vi "Write and Read Multiple Registers Response.vi"(8 "error in (no error)":errorcluster, 10 "Modbus data unit in":refnum<class "Modbus Data Unit (PDU).lvclass">) -> (0 "error out":errorcluster, 1 "registers":u16[](array[numeric]), 2 "byte count":u8)   [LabVIEW 2017, in "SubVIs.lvlib" / "Master Function Definition.lvlib"]
doc: "Decodes the response generated by the write and read multiple holding registers function."
uses:
  <vilib>/Modbus/subvis/Data and Functions/Master Function Definition/Master Function Definition.lvlib
  <vilib>/Modbus/subvis/Modbus Data Unit (PDU)/Modbus Data Unit (PDU).lvclass
  <vilib>/Modbus/subvis/SubVIs.lvlib
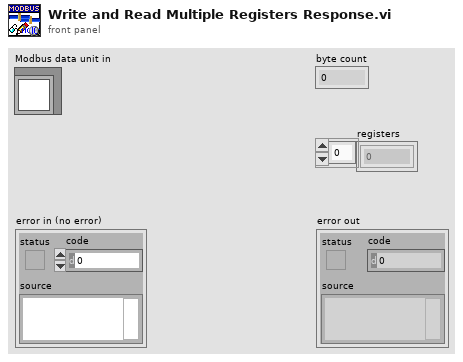
[diagram p1: front panel]
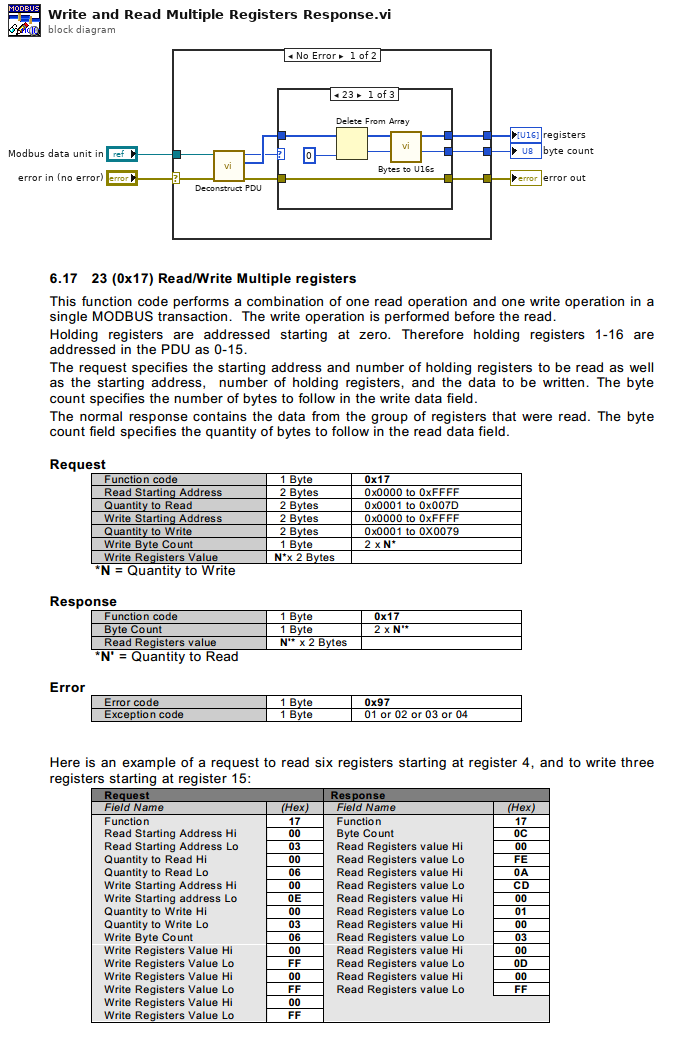
[diagram p0: block diagram]
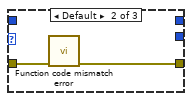
[diagram p2: hidden frame]
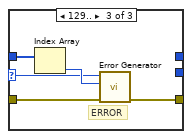
[diagram p3: hidden frame]
diagram:
  n1 = case shown="No Error" "error in (no error)" {
    selector: "error in (no error)" -> [w12 w27]
    tunnel: [w13 w27] -> w4
    tunnel: "Modbus data unit in" -> [w10 _]
    tunnel: [w7 _] -> w2
    tunnel: [w6 _] -> w1
    frame No Error {
      n2 = call <vilib>:"Deconstruct PDU.vi"("error in (no error)"=w12, "Modbus data unit in"=w10) -> ("error out"=w9:errorcluster, "data"=w11:u8[], "function"=w8:u8)  [unwired: 7 in]
      n3 = case shown="23" w8 {
        selector: w8 -> [_ _ w22]
        tunnel: w9 -> [w19 w21 w23]
        tunnel: w11 -> [w16 _ w26]
        tunnel: [w19 w20 w25] -> w13
        tunnel: [w15 _ _] -> w7
        tunnel: [w14 _ _] -> w6
        frame 23 {
          n4 = Delete From Array(array=w16, index=0) -> (deleted portion=w15:u8, array with subset deleted=w17:u8[])  [unwired: 1 in]
          n5 = call <vilib>:"Bytes to U16s.vi"("bytes"=w17) -> ("registers"=w14:u16[])  [unwired: 10 in]
        }
        frame Default {
          n6 = call <vilib>:"Function code mismatch error.vi"("error in (no error)"=w21) -> ("error out"=w20:errorcluster)  [unwired: 10 in]
        }
        frame 129.. {
          # "ERROR"
          n7 = Index Array(array=w26) -> (element=w24:u8)  [unwired: 1 in]
          n8 = call <vilib>:"Error Generator.vi"("error in (no error)"=w23, "data return (error code)"=w24, "function return"=w22) -> ("error out"=w25:errorcluster)  [unwired: 8 in]
        }
      }
    }
    frame Error {
    }
  }
  "error out" <- w4
  "byte count" <- w2
  "registers" <- w1
